vi "Conf Trigger.vi"(0 "VISA Resource Name":refnum<visa-resource-name>, 1 "Set/Check (F:Set)":bool, 2 "Check Parameter(0:Source)":T3(ring), 3 "Wait for Trigger? (F:No)":bool, 5 "Source (1:Immediate)":T2(ring)=enum."Immediate", 7 "Time-Scan Interval (1:Min)":enum16{"Manual", "Minimum", "Maximum"}(ring)=enum."Minimum", 9 "Interval Value (0)":dbl min=0.0 max=359999.0 format="%.2f", 11 "error in (no error)":errorcluster, 12 "Max Trigger Count (3:Inf)":T1(ring)=enum."Infinity", 13 "# Triggers (1)":u16=1 min=1 max=50000 step=1) -> (4 "VISA Resource Name Out":refnum<visa-resource-name>, 8 "Configuration ?":string, 15 "error out":errorcluster)   [LabVIEW 2012, in "Agilent 34970.lvlib"]
doc: "This VI lets you configure the instrument's triggering parameters. For example, you can set the trigger source, scan interval, etc.\n\nAfter configuration, you can put the instrument into \"wait for trigger\" mode."
uses:
  <instrlib>/Agilent 34970/Agilent 34970.lvlib
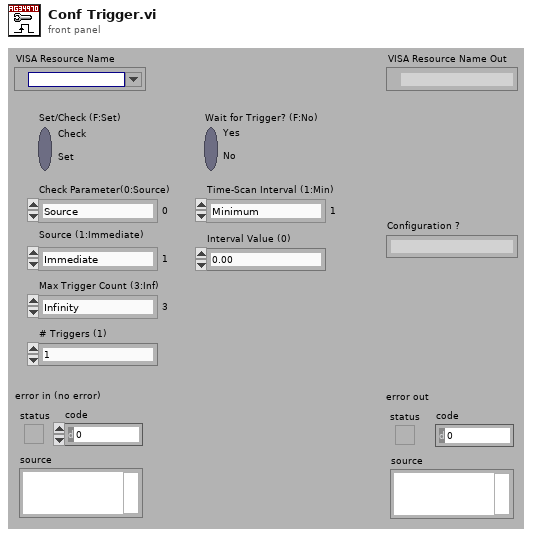
[diagram p1: front panel]
types:
  T1 = enum16{"Manual", "Minimum", "Maximum", "Infinity"}
  T2 = enum16{"Bus", "Immediate", "External", "Alarm 1", "Alarm 2", "Alarm 3", "Alarm 4", "Timer"}
  T3 = enum16{"Source", "Scan-Scan Interval", "Max Trigger Count"}
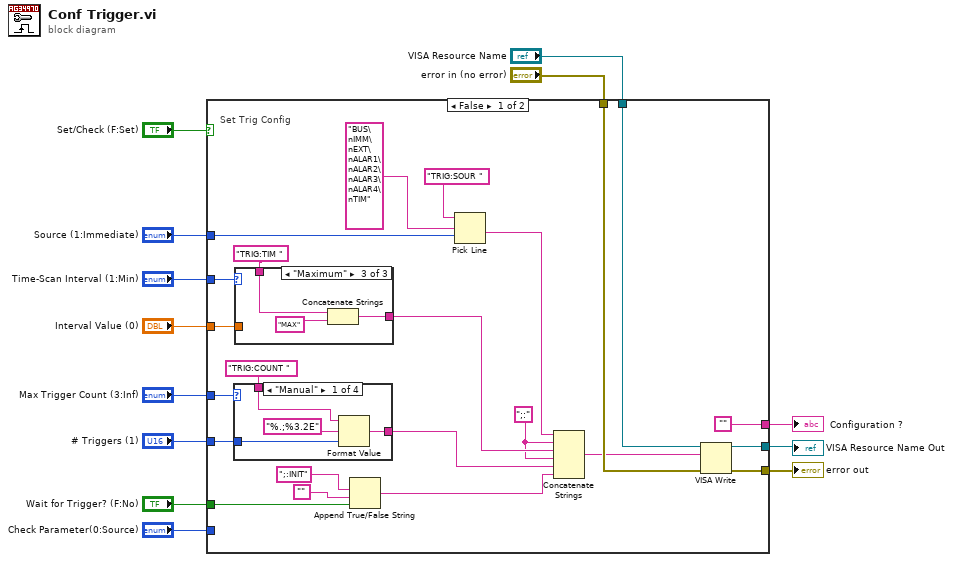
[diagram p0: block diagram]
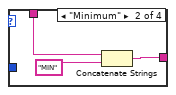
[diagram p2: hidden frame]
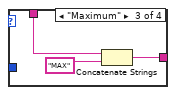
[diagram p3: hidden frame]
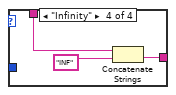
[diagram p4: hidden frame]
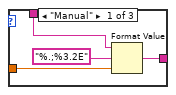
[diagram p5: hidden frame]
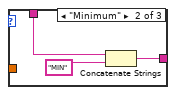
[diagram p6: hidden frame]
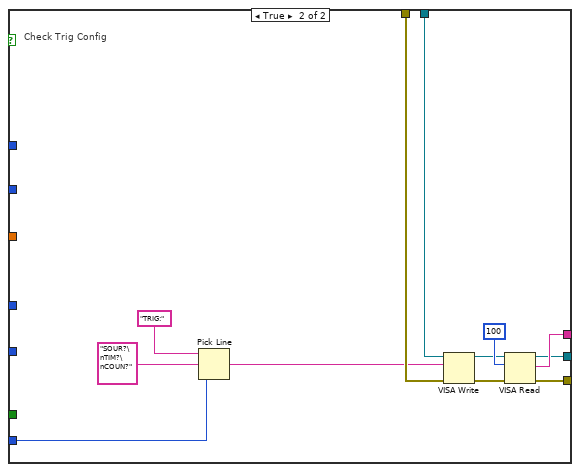
[diagram p7: hidden frame]
diagram:
  n1 = case shown="False" "Set/Check (F:Set)" {
    tunnel: [w32 w71] -> w3
    tunnel: [w33 w68] -> w4
    tunnel: ["" w69] -> w12
    tunnel: "VISA Resource Name" -> [w35 w67]
    tunnel: "error in (no error)" -> [w34 w66]
    tunnel: "Check Parameter(0:Source)" -> [_ w61]
    tunnel: "Source (1:Immediate)" -> [w29 _]
    tunnel: "Time-Scan Interval (1:Min)" -> [w28 _]
    tunnel: "Interval Value (0)" -> [w26 _]
    tunnel: "Max Trigger Count (3:Inf)" -> [w24 _]
    tunnel: "# Triggers (1)" -> [w23 _]
    tunnel: "Wait for Trigger? (F:No)" -> [w15 _]
    frame False {
      w20 = ";:"
      # "Set Trig Config"
      n2 = case shown="\"Manual\"" w24 {
        tunnel: "TRIG:COUNT " -> [w39 w43 w45 w48]
        tunnel: [w38 w41 w44 w47] -> w19
        tunnel: w23 -> [w37 _ _ _]
        frame "Manual" {
          n3 = Format Value(string ("")=w39, format string="%.;%3.2E", value (0)=w37) -> (output string=w38:string)
        }
        frame "Minimum" {
          n4 = Concatenate Strings(w43, "MIN") -> (w41:string)
        }
        frame "Maximum" {
          n5 = Concatenate Strings(w45, "MAX") -> (w44:string)
        }
        frame "Infinity" {
          n6 = Concatenate Strings(w48, "INF") -> (w47:string)
        }
      }
      n7 = case shown="\"Maximum\"" w28 {
        tunnel: "TRIG:TIM " -> [w52 w56 w58]
        tunnel: w26 -> [w51 _ _]
        tunnel: [w50 w54 w57] -> w21
        frame "Manual" {
          n8 = Format Value(string ("")=w52, format string="%.;%3.2E", value (0)=w51) -> (output string=w50:string)
        }
        frame "Minimum" {
          n9 = Concatenate Strings(w56, "MIN") -> (w54:string)
        }
        frame "Maximum" {
          n10 = Concatenate Strings(w58, "MAX") -> (w57:string)
        }
      }
      n11 = Append True/False String(1:w15, 2:"", 3:";:INIT" ("true string")) -> (0:w14:string)  [unwired: 1 in]
      n12 = Pick Line(string ("")="TRIG:SOUR ", multi-line string="BUS\nIMM\nEXT\nALAR1\nALAR2\nALAR3\nALAR4\nTIM", line index=w29) -> (output string=w22:string)
      n13 = Concatenate Strings(w22, w20, w21, w20, w19, w14) -> (w18:string)
      n14 = VISA Write(VISA resource name=w35, write buffer=w18, error in (no error)=w34) -> (VISA resource name out=w33:refnum<visa-resource-name>, error out=w32:errorcluster)  [unwired: 1 out]
    }
    frame True {
      # "Check Trig Config"
      n15 = Pick Line(string ("")="TRIG:", multi-line string="SOUR?\nTIM?\nCOUN?", line index=w61) -> (output string=w60:string)
      n16 = VISA Write(VISA resource name=w67, write buffer=w60, error in (no error)=w66) -> (VISA resource name out=w65:refnum<visa-resource-name>, error out=w64:errorcluster)  [unwired: 1 out]
      n17 = VISA Read(VISA resource name=w65, byte count=u32 100 ("byte count (0)"), error in (no error)=w64) -> (VISA resource name out=w68:refnum<visa-resource-name>, read buffer=w69:string, error out=w71:errorcluster)  [unwired: 1 out]
    }
  }
  "Configuration ?" <- w12
  "VISA Resource Name Out" <- w4
  "error out" <- w3
